vi "SetToRandomPosition.vi"(8 "error in (no error)":errorcluster, 10 "SnakeGame in":refnum<class "SnakeGame.lvclass">, 11 "SnakeSwitch in":refnum<class "SnakeSwitch.lvclass">) -> (0 "error out":errorcluster, 2 "SnakeGame out":refnum<class "SnakeGame.lvclass">, 3 "SnakeSwitch out":refnum<class "SnakeSwitch.lvclass">)   [LabVIEW 2019, in "RT_Game.lvlib" / "SnakeSwitch.lvclass"]
uses:
  SnakeSwitch.lvclass
  C:/Users/FreshBob/Dropbox/VIs/myRIO_GameConsole/RT/RT_Game/GameObject/GameObject.lvclass
  SnakeGame/SnakeGame.lvclass
  GameObject/GameObject.lvclass/GameObject.ctl
  SnakeSwitch.lvclass/SnakeSwitch.ctl
  GameObject/Write position.vi
  GameObject/Write IsActive.vi
  Read Tilecode.vi
  GameObject/Read IsActive.vi
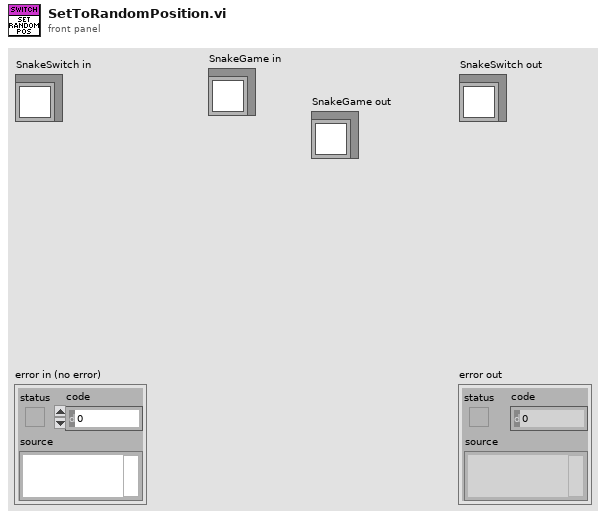
[diagram p1: front panel]
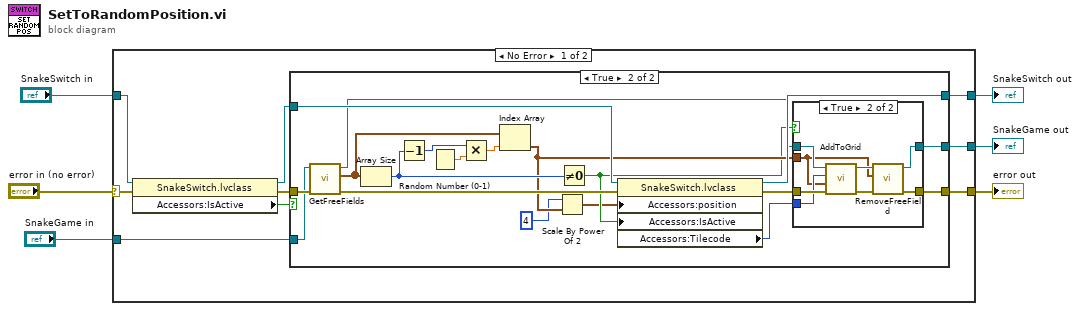
[diagram p0: block diagram]
diagram:
  n1 = case shown="No Error" "error in (no error)" {
    selector: "error in (no error)" -> [w14 w50]
    tunnel: [w12 w50] -> w5
    tunnel: [w15 w49] -> w3
    tunnel: "SnakeSwitch in" -> [w9 w49]
    tunnel: "SnakeGame in" -> [w13 w48]
    tunnel: [w11 w48] -> w1
    frame No Error {
      n2 = property class="SnakeSwitch.lvclass"(reference=w9, error in=w14) -> (reference out=w8:refnum<class "SnakeSwitch.lvclass">, error out=w10:errorcluster, "Accessors:IsActive"=w7:bool)
      n3 = case shown="True" w7 {
        tunnel: w8 -> [w18 w27]
        tunnel: [w18 w36] -> w15
        tunnel: w10 -> [w16 w28]
        tunnel: w13 -> [w17 w26]
        tunnel: [w16 w25] -> w12
        tunnel: [w17 w24] -> w11
        frame False {
        }
        frame True {
          n4 = call "GetFreeFields.vi"("error in (no error)"=w28, "SnakeGame in"=w26) -> ("error out"=w35:errorcluster, "FreeFields"=w31:cluster{i16, i16}[], "SnakeGame out"=w21:refnum<class "SnakeGame.lvclass">)  [unwired: 7 in]
          n5 = Array Size(array=w31) -> (size(s)=w30:i32)
          n6 = Decrement(x=w30) -> (x-1=w33:i32)
          n7 = Random Number (0-1)() -> (number: 0 to 1=w34:dbl)
          n8 = Multiply(x=w33, y=w34) -> (x*y=w32:dbl)
          n9 = Index Array(array=w31, index=w32) -> (element=w23:cluster{i16, i16})
          n10 = Scale By Power Of 2(n=i16 4, x=w23) -> (x*2^n=w20:cluster{i16, i16})
          n11 = Not Equal To 0?(x=w30) -> (x != 0?=w22:bool)
          n12 = property class="SnakeSwitch.lvclass"(reference=w27, error in=w35, "Accessors:position"=w20, "Accessors:IsActive"=w22) -> (reference out=w36:refnum<class "SnakeSwitch.lvclass">, error out=w37:errorcluster, "Accessors:Tilecode"=w29:u32)
          n13 = case shown="True" w22 {
            tunnel: w37 -> [w38 w47]
            tunnel: w21 -> [w39 w45]
            tunnel: w29 -> [_ w44]
            tunnel: [w38 w43] -> w25
            tunnel: [w39 w41] -> w24
            tunnel: w23 -> [_ w40]
            frame False {
            }
            frame True {
              n14 = call "AddToGrid.vi"("error in (no error)"=w47, "Coordinate"=w40, "Tilecode"=w44, "SnakeGame in"=w45) -> ("error out"=w46:errorcluster, "SnakeGame out"=w42:refnum<class "SnakeGame.lvclass">)  [unwired: 6 in]
              n15 = call "RemoveFreeField.vi"("error in (no error)"=w46, "Coordinate"=w40, "SnakeGame in"=w42) -> ("error out"=w43:errorcluster, "SnakeGame out"=w41:refnum<class "SnakeGame.lvclass">)  [unwired: 7 in]
            }
          }
        }
      }
    }
    frame Error {
    }
  }
  "error out" <- w5
  "SnakeSwitch out" <- w3
  "SnakeGame out" <- w1
